vi "test12.1-SyncMessage_Event.vi"(8 "error in (no error)":errorcluster, 11 "TestCase in":refnum<class "testcase-CSMGlobalLog.lvclass">) -> (0 "error out":errorcluster, 3 "TestCase out":refnum<class "testcase-CSMGlobalLog.lvclass">)   [LabVIEW 2017, in "testcase-CSMGlobalLog.lvclass"]
uses:
  testcase-CSMGlobalLog.lvclass
  testcase-CSMGlobalLog.lvclass/testcase-CSMGlobalLog.ctl
  src/user.lib/_NEVSTOP/Communicable State Machine(CSM)/_Support/Typedef/_CSM_GlobalLog_MSG.ctl
  src/user.lib/_NEVSTOP/Communicable State Machine(CSM)/_Support/Typedef/_CSM_Response Source Message.ctl
  src/user.lib/_NEVSTOP/Communicable State Machine(CSM)/_Support/Typedef/_CSM_GlobalLog_MSG_TYPE.ctl
  c0dc643a-0362-49fc-99f4-5251266ba5a0.vi
  src/user.lib/_NEVSTOP/Communicable State Machine(CSM)/_Support/GlobalEvent/GEvt-Generate with Rule Check.vi
  src/user.lib/_NEVSTOP/Communicable State Machine(CSM)/AdvanceAPI/CSM - Convert Error to Argument.vi
  src/user.lib/_NEVSTOP/Communicable State Machine(CSM)/AdvanceAPI/CSM - Make String Arguments Safe.vi
  src/user.lib/_NEVSTOP/Communicable State Machine(CSM)/AdvanceAPI/CSM - Keywords.vi
  src/user.lib/_NEVSTOP/Communicable State Machine(CSM)/_Support/GlobalEvent/Cache-GEvt Refs.vi
  src/user.lib/_NEVSTOP/Communicable State Machine(CSM)/_Support/GlobalEvent/LogFilter/LogFilter - Check.vi
  src/user.lib/_NEVSTOP/Communicable State Machine(CSM)/_Support/GlobalEvent/LogFilter/LogFilter.lvclass
  <vilib>/addons/_JKI Toolkits/VI Tester/TestCase.llb/TestCase.lvclass
  src/user.lib/_NEVSTOP/Communicable State Machine(CSM)/Communicable State Machine.lvlib
  CSM/CSM-Testcase.lvlib
  C:/Program Files (x86)/National Instruments/LabVIEW 2017/vi.lib/addons/_JKI Toolkits/VI Tester/TestCase.llb/TestCase.lvclass
panel:
  out "String cache each loop":string
  out "LoopCount":i32
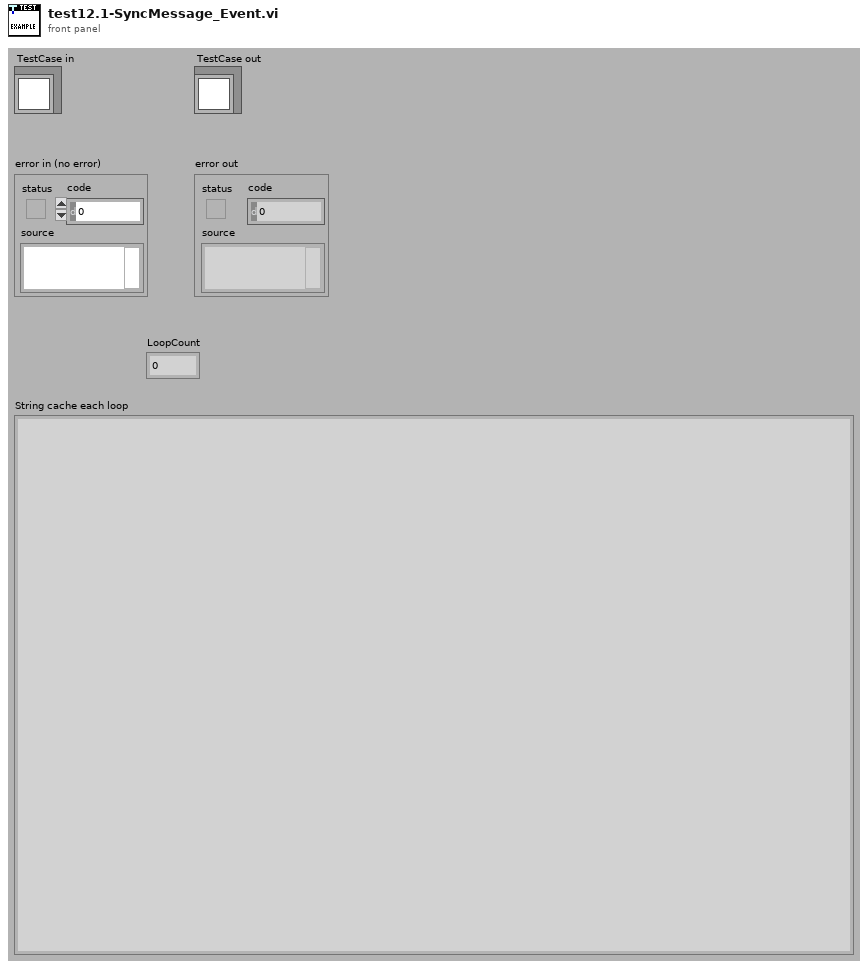
[diagram p1: front panel]
types:
  T1 = typedef "Communicable State Machine.lvlib/_CSM_GlobalLog_MSG.ctl" = cluster{"Name (\"\" to Use UUID)":string, "Current State":string, "Arguments":string, "Source Message":T2, "Source Module":string, "Complete(T)/Start(F)":bool, "LogType":T3, "Time Stamp":timestamp}
  T2 = typedef "Communicable State Machine.lvlib/_CSM_Response Source Message.ctl" = cluster{"‘State":string, "’Arguments":string, "’Error":errorcluster}
  T3 = typedef "Communicable State Machine.lvlib/_CSM_GlobalLog_MSG_TYPE.ctl" = enum16{"User Log", "State Change", "Status", "Interrupt", "Register", "Unregister", "Error Log", "Module Created", "Module Destroyed", "Async Message", "No-Rep Async Message", "Sync Message"}
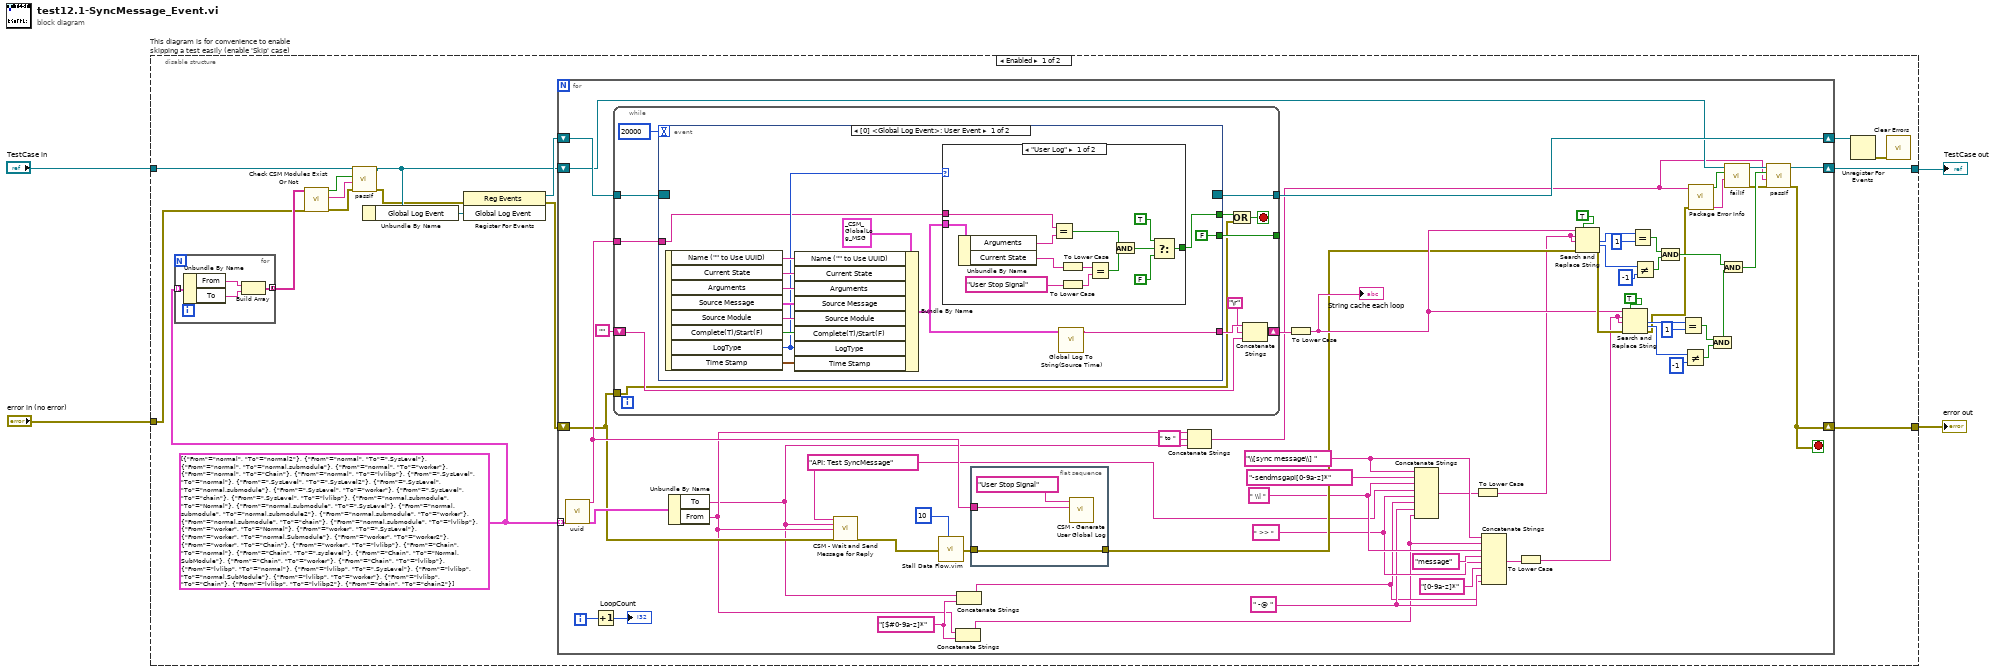
[diagram p0: block diagram]
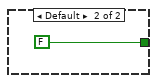
[diagram p2: hidden frame]
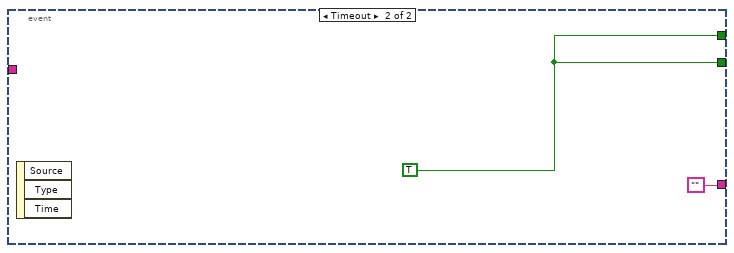
[diagram p3: hidden frame]
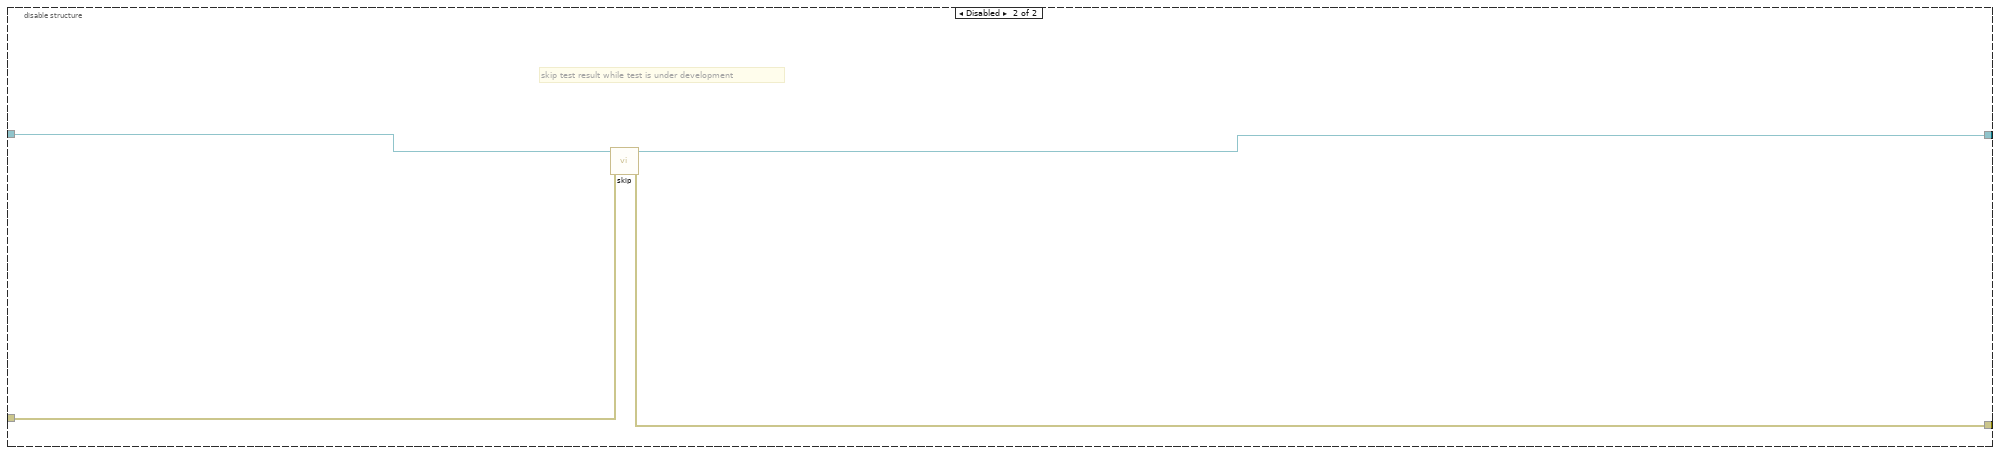
[diagram p4: hidden frame]
diagram:
  n1 = disable-structure "This diagram is for convenience to enable skipping a test easily (enable 'Skip' case)" shown="Enabled" {
    disable-tunnel: "TestCase in" -> [w8 w132]
    disable-tunnel: [w16 w130] -> w1
    disable-tunnel: [w15 w131] -> w3
    disable-tunnel: "error in (no error)" -> [w9 w129]
    frame Enabled {
      w10 = cluster{"From":string, "To":string}[] [{"From"="normal", "To"="normal2"}, {"From"="normal", "To"=".SysLevel"}, {"From"="normal", "To"="normal.submodule"}, {"From"="normal", "To"="worker"}, {"From"="normal", "To"="Chain"}, {"From"="normal", "To"="lvlibp"}, {"From"=".SysLevel", "To"="normal"}, {"From"=".SysLevel", "To"=".SysLevel2"}, {"From"=".SysLevel", "To"="normal.submodule"}, {"From"=".SysLevel", "To"="worker"}, {"From"=".SysLevel", "To"="chain"}, {"From"=".SysLevel", "To"="lvlibp"}, {"From"="normal.submodule", "To"="Normal"}, {"From"="normal.submodule", "To"=".SysLevel"}, {"From"="normal.submodule", "To"="normal.submodule2"}, {"From"="normal.submodule", "To"="worker"}, {"From"="normal.submodule", "To"="chain"}, {"From"="normal.submodule", "To"="lvlibp"}, {"From"="worker", "To"="Normal"}, {"From"="worker", "To"=".SysLevel"}, {"From"="worker", "To"="normal.Submodule"}, {"From"="worker", "To"="worker2"}, {"From"="worker", "To"="Chain"}, {"From"="worker", "To"="lvlibp"}, {"From"="Chain", "To"="normal"}, {"From"="Chain", "To"=".syslevel"}, {"From"="Chain", "To"="Normal.SubModule"}, {"From"="Chain", "To"="worker"}, {"From"="Chain", "To"="lvlibp"}, {"From"="lvlibp", "To"="normal"}, {"From"="lvlibp", "To"=".SysLevel"}, {"From"="lvlibp", "To"="normal.SubModule"}, {"From"="lvlibp", "To"="worker"}, {"From"="lvlibp", "To"="Chain"}, {"From"="lvlibp", "To"="lvlibp2"}, {"From"="chain", "To"="chain2"}]
      n2 = for {
        tunnel: w10 -> [w24] mode=indexing
        tunnel: [w21] -> w12 mode=concatenating
        n3 = Unbundle By Name(w24) -> ("From"=w23:string, "To"=w22:string)
        n4 = Build Array(w23, w22) -> (w21:string[])
      }
      n5 = call "Check CSM Modules Exist Or Not.vi"("error in"=w9, "CSM names in"=w12) -> ("error out"=w14:errorcluster, "Debug string"=w13:string, "All Modules Exist?"=w11:bool)  [unwired: 7 in]
      n6 = call-dynamic "passIf.vi"("error in (no error)"=w14, "message (\"\")"=w13, "pass"=w11, "TestCase in"=w8) -> ("error out"=w6:errorcluster, "TestCase out"=w7:refnum<class "testcase-CSMGlobalLog.lvclass">)  [unwired: 6 in]
      n7 = Unbundle By Name(w7) -> ("Global Log Event"=w20:refnum<user-event>)
      n8 = register-events(error in=w6, w20) -> (reference out=w19:refnum<event-registration>, error out=w17:errorcluster)  [unwired: 1 in]
      n9 = for {
        shift-right: [w82] -> w18
        shift-left: w19 -> [w83]
        shift-right: [w79] -> w15
        shift-left: w17 -> [w35]
        tunnel: w10 -> [w60] mode=indexing
        shift-right: [w81] -> w16
        shift-left: w7 -> [w33]
        i -> [w57]
        stop <- w79 stop-if-true
        w38 = "[$#0-9a-z]*" ("string")
        w44 = " -@ "
        w46 = " >> "
        w48 = " \\| "
        w49 = "\\[sync message\\] "
        w41 = "API: Test SyncMessage" ("State")
        n10 = call "uuid.vi"() -> ("UUID"=w58:string)  [unwired: 11 in]
        n11 = Increment(x=w57) -> (x+1=→"LoopCount":i32)
        n12 = while {
          tunnel: w83 -> [w98]
          tunnel: [w97] -> w82
          shift-right: [w90] -> w51
          shift-left: "" -> [w93]
          tunnel: w58 -> [w95]
          tunnel: [w94] -> _
          tunnel: w35 -> [w87]
          stop <- w89 stop-if-true
          n13 = event shown="[0] <Global Log Event>: User Event" {
            selector: w98 -> [_ _]
            dyn-events: [_ _] -> w97
            timeout: 20000 -> [_ _]
            tunnel: [w99 ""] -> w92
            tunnel: [w101 w128] -> w88
            tunnel: w95 -> [w102 _]
            tunnel: [FALSE ("Stop") w128] -> w94
            event User Event {
              n14 = event-data() -> ("Name (\"\" to Use UUID)"=w111:string, "Current State"=w110:string, "Arguments"=w109:string, "Source Message"=w108:T2, "Source Module"=w107:string, "Complete(T)/Start(F)"=w106:bool, "LogType"=w103:T3, "Time Stamp"=w105:timestamp)  [unwired: 1 in]
              n15 = Bundle By Name(cluster=T1 {"Name (\"\" to Use UUID)"="", "Current State"="", "Arguments"="", "Source Message"={"‘State"="", "’Arguments"="", "’Error"={"status"=FALSE, "code"=0, "source"=""}}, "Source Module"="", "Complete(T)/Start(F)"=FALSE, "LogType"=enum."State Change", "Time Stamp"=timestamp(0 s since 1904-01-01)} ("Cross CSM Data"), "Name (\"\" to Use UUID)"=w111, "Current State"=w110, "Arguments"=w109, "Source Message"=w108, "Source Module"=w107, "Complete(T)/Start(F)"=w106, "LogType"=w103, "Time Stamp"=w105) -> (w100:T1)
              n16 = case shown="\"User Log\"" w103 {
                tunnel: w100 -> [w125 _]
                tunnel: w102 -> [w124 _]
                tunnel: [w113 FALSE] -> w101
                frame "User Log" {
                  n17 = Unbundle By Name(w125) -> ("Arguments"=w123:string, "Current State"=w122:string)
                  n18 = Equal?(x=w124, y=w123) -> (x = y?=w117:bool)
                  n19 = To Lower Case(string=w122) -> (all lower case string=w121:string)
                  n20 = To Lower Case(string="User Stop Signal" ("Log")) -> (all lower case string=w119:string)
                  n21 = Equal?(x=w121, y=w119) -> (x = y?=w118:bool)
                  n22 = And(x=w117, y=w118) -> (x .and. y?=w116:bool)
                  n23 = Select(t=TRUE, s=w116, f=FALSE) -> (s? t:f=w113:bool)
                }
                frame Default {
                }
              }
              n24 = call "Global Log To String(Source Time).vi"("Log"=w100) -> ("Log String"=w99:string)  [unwired: 9 in]
            }
            event Timeout {
              w128 = TRUE ("Stop")
              n25 = event-data() -> ()  [unwired: 1 in, 3 out]
            }
          }
          n26 = Or(x=w88, y=w87) -> (x .or. y?=w89:bool)
          n27 = Concatenate Strings(w92, "\r", w93) -> (w90:string)
        }
        n28 = Unbundle By Name(w60) -> ("To"=w27:string, "From"=w28:string)
        n29 = call "CSM - Wait and Send Message for Reply.vi"("State"=w41, "Arguments (\"\")"=w27, "Target Module"=w28, "Error In (No Error)"=w35) -> ("error out"=w54:errorcluster)  [unwired: 8 in, 3 out]
        n30 = call "Stall Data Flow.vim"("value in"=w54, "milliseconds to wait"=u32 10) -> ("value out"=w59:errorcluster)  [unwired: 1 out]
        n31 = Concatenate Strings(w28, w38) -> (w36:string)
        n32 = Concatenate Strings(w27, w38) -> (w37:string)
        n33 = flat-sequence {
          tunnel: w58 -> [w85]
          tunnel: w59 -> [w84]
          tunnel: [w84] -> w52
          frame #0 {
            n34 = call "CSM - Generate User Global Log.vi"("Arguments"=w85, "Log"="User Stop Signal") -> ()  [unwired: 9 in, 1 out]
          }
        }
        n35 = Concatenate Strings(w28, " to " ("string"), w27) -> (w25:string)
        n36 = To Lower Case(string=w51) -> (all lower case string=w53:string)
        "String cache each loop" <- w53
        n37 = Concatenate Strings(w49, "-sendmsgapi[0-9a-z]*", w48, w41, w46, w37, w44, w36) -> (w43:string)
        n38 = To Lower Case(string=w43) -> (all lower case string=w40:string)
        n39 = Concatenate Strings(w49, w36, w48, "message", w46, "[0-9a-z]*", w44, w37) -> (w42:string)
        n40 = To Lower Case(string=w42) -> (all lower case string=w39:string)
        n41 = Search and Replace String(replace all?=TRUE ("replace all? (F)"), input string=w53, search string=w40, replace string=w40, error in=w52) -> (number of replacements=w68:i32, offset past replacement=w69:i32, error out=w76:errorcluster)  [unwired: 3 in, 1 out]
        n42 = Search and Replace String(replace all?=TRUE ("replace all? (F)"), input string=w53, search string=w39, replace string=w39, error in=w76) -> (number of replacements=w75:i32, offset past replacement=w74:i32, error out=w29:errorcluster)  [unwired: 3 in, 1 out]
        n43 = Equal?(x=w68, y=1) -> (x = y?=w70:bool)
        n44 = Not Equal?(x=w69, y=-1) -> (x != y?=w71:bool)
        n45 = And(x=w70, y=w71) -> (x .and. y?=w78:bool)
        n46 = Equal?(x=w75, y=1) -> (x = y?=w73:bool)
        n47 = Not Equal?(x=w74, y=-1) -> (x != y?=w72:bool)
        n48 = call "Package Error Info.vi"("error in"=w29, "String in"=w25) -> ("packed error info out"=w30:string, "error status"=w34:bool)  [unwired: 8 in]
        n49 = And(x=w73, y=w72) -> (x .and. y?=w77:bool)
        n50 = And(x=w78, y=w77) -> (x .and. y?=w56:bool)
        n51 = call-dynamic "failIf.vi"("message (\"\")"=w30, "fail"=w34, "TestCase in"=w33) -> ("error out"=w31:errorcluster, "TestCase out"=w32:refnum<class "testcase-CSMGlobalLog.lvclass">)  [unwired: 7 in]
        n52 = call-dynamic "passIf.vi"("error in (no error)"=w31, "message (\"\")"=w25, "pass"=w56, "TestCase in"=w32) -> ("error out"=w79:errorcluster, "TestCase out"=w81:refnum<class "testcase-CSMGlobalLog.lvclass">)  [unwired: 6 in]
      }
      n53 = Unregister For Events(event registration refnum=w18) -> (error out=w5:errorcluster)  [unwired: 1 in]
      n54 = call <vilib>:"Clear Errors.vi"("error in (no error)"=w5) -> ()  [unwired: 5 in, 2 out]
    }
    frame Disabled {
      # "skip test result while test is under development"
      n55 = call <vilib>:"skip.vi"("error in (no error)"=w129, "TestCase in"=w132) -> ("error out"=w131:errorcluster, "TestCase out"=w130:refnum<class "testcase-CSMGlobalLog.lvclass">)  [unwired: 8 in]
    }
  }
  "error out" <- w3
  "TestCase out" <- w1
